vi "test_scd_dataToCluster.vi"(8 "error in (no error)":errorcluster) -> (0 "error out":errorcluster)   [LabVIEW 2023, in "horiba.test.lvlib"]
uses:
  horiba.test.lvlib
  Classes/SCD/scdData.ctl
  3f95e01c-6737-415e-b7d2-11fb20076c28.vi
  <vilib>/JDP Science/JSONtext/JSON text to Variant.vi
  <vilib>/addons/_JKI Toolkits/Caraya/classes/Assert/Assert Equal Value_Variant.vi
  <vilib>/addons/_JKI Toolkits/Caraya/classes/Assert/Assert Not Error.vi
  <vilib>/JDP Science/JSONtext/LVClass Serializer/JSONtext LVClass Serializer.lvclass
  <vilib>/addons/_JKI Toolkits/Caraya/classes/Test/Test.lvclass
  <vilib>/addons/_JKI Toolkits/Caraya/classes/Assert/Assert.lvclass
  Classes/SCD/SCD.lvclass
panel:
  # "Connector Pane"
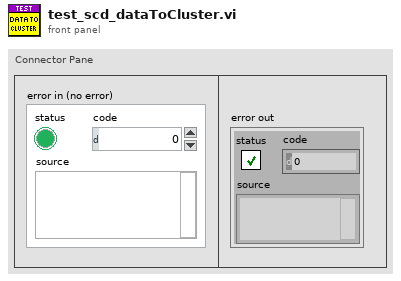
[diagram p1: front panel]
types:
  T1 = typedef "horiba.lvlib/SCD.lvclass/scdData.ctl" = cluster{"data":cluster{"currentSignal":cluster{"unit":string, "value":dbl}, "elapsedTime":dbl, "event_marker":bool, "overscale_current_channel":bool, "overscale_voltage_channel":bool, "pmtSignal":cluster{"unit":string, "value":dbl}, "pointNumber":dbl, "ppdSignal":cluster{"unit":string, "value":dbl}, "voltageSignal":cluster{"unit":string, "value":dbl}}[]}
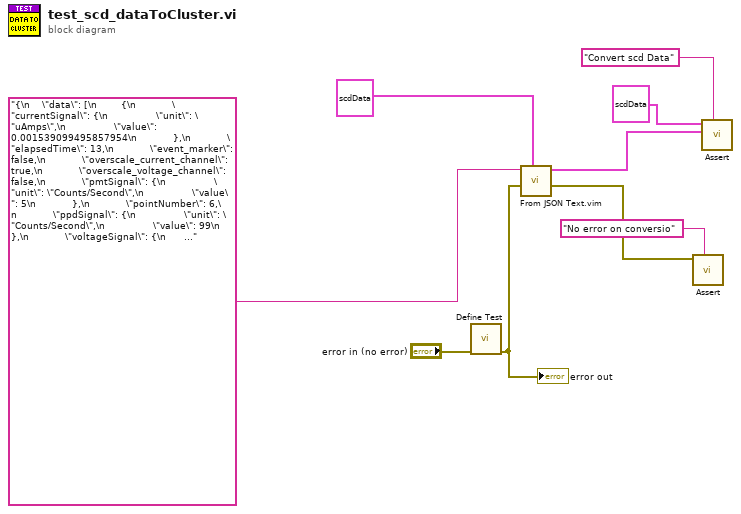
[diagram p0: block diagram]
diagram:
  n1 = call <vilib>:"Define Test.vi"("error in (no error)"="error in (no error)") -> ("error out"=w2:errorcluster)  [unwired: 9 in, 1 out]
  "error out" <- w2
  n2 = call "From JSON Text.vim"("Data Type and Default Value"=T1 {"data"=[{"currentSignal"={"unit"="", "value"=0.0}, "elapsedTime"=0.0, "event_marker"=FALSE, "overscale_current_channel"=FALSE, "overscale_voltage_channel"=FALSE, "pmtSignal"={"unit"="", "value"=0.0}, "pointNumber"=0.0, "ppdSignal"={"unit"="0", "value"=0.0}, "voltageSignal"={"unit"="", "value"=0.0}}]} ("scdData"), "error in (no error)"=w2, "JSON"="{\n    \"data\": [\n        {\n            \"currentSignal\": {\n                \"unit\": \"uAmps\",\n                \"value\": 0.001539099495857954\n            },\n            \"elapsedTime\": 13,\n            \"event_marker\": false,\n            \"overscale_current_channel\": true,\n            \"overscale_voltage_channel\": false,\n            \"pmtSignal\": {\n                \"unit\": \"Counts/Second\",\n                \"value\": 5\n            },\n            \"pointNumber\": 6,\n            \"ppdSignal\": {\n                \"unit\": \"Counts/Second\",\n                \"value\": 99\n            },\n            \"voltageSignal\": {\n                \"unit\": \"Volts\",\n                \"value\": -0.0006916072452440858\n            }\n        }\n    ]\n}") -> ("error out"=w3:errorcluster, "Data out"=w4:T1)  [unwired: 7 in]
  n3 = call-poly <vilib>:"Assert.vi"("Label"="No error on conversio", "Not Error?"=w3) -> ()  [unwired: 8 in, 2 out]
  n4 = call-poly <vilib>:"Assert.vi"("Label"="Convert scd Data" ("Label (VI Title)"), "Y"=w4, "X"=T1 {"data"=[{"currentSignal"={"unit"="uAmps", "value"=0.001539099495857954}, "elapsedTime"=13.0, "event_marker"=FALSE, "overscale_current_channel"=TRUE, "overscale_voltage_channel"=FALSE, "pmtSignal"={"unit"="Counts/Second", "value"=5.0}, "pointNumber"=6.0, "ppdSignal"={"unit"="Counts/Second", "value"=99.0}, "voltageSignal"={"unit"="Volts", "value"=-0.0006916072452440858}}]} ("Data out")) -> ()  [unwired: 7 in, 2 out]
